vi "Verify Scripting Code.Caraya.vi"(8 "error in":errorcluster) -> (0 "error out":errorcluster)   [LabVIEW 2026, in "Caraya Extension Tests.lvclass"]
uses:
  Caraya Extension Tests.lvclass
  Source/Approval Tests/Options/Options.lvclass
  <vilib>/addons/_JKI Toolkits/Caraya/classes/Test/Test.lvclass
  Source/Extensions/Caraya.Extension/Caraya.Extension.lvlib
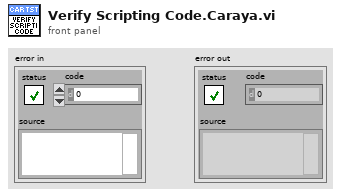
[diagram p1: front panel]
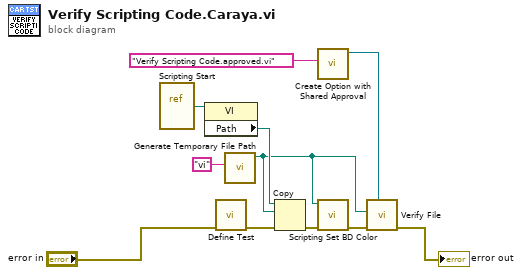
[diagram p0: block diagram]
diagram:
  n1 = vi-ref "Scripting Start.vi"() -> (w6:refnum<vi>)
  n2 = property on="Property Node" class="VI"(reference=w6) -> ("Path"=w4:path)  [unwired: 1 in, 2 out]
  n3 = call <vilib>:"Define Test.vi"("error in (no error)"="error in") -> ("error out"=w8:errorcluster)  [unwired: 9 in, 1 out]
  n4 = call <vilib>:"Generate Temporary File Path.vi"("Temporary File Extension (tmp)"="vi") -> ("Unique Temporary File Path"=w3:path)  [unwired: 9 in, 1 out]
  n5 = Copy(8:w8, 10:w3, 11:w4) -> (0:w7:errorcluster)  [unwired: 2 in, 2 out]
  n6 = call "Create Option with Shared Approval.vi"("Filename"="Verify Scripting Code.approved.vi") -> ("Options outs"=w1:refnum<class "Options.lvclass">)  [unwired: 10 in]
  n7 = call "Scripting Set BD Color.vi"("error in"=w7, "Path"=w3) -> ("error out"=w9:errorcluster)  [unwired: 9 in]
  n8 = call "Verify File.vi"("Options"=w1, "error in"=w9, "path to file"=w3) -> ("error out"=→"error out":errorcluster)  [unwired: 7 in, 1 out]
